vi "common_map_read.vi"(8 "error in":errorcluster, 11 "file path":path) -> (0 "error out":errorcluster, 3 "common map":map{string, T1}(c390))   [LabVIEW 2024, in "MemoryManager.lvclass"]
uses:
  MemoryManager.lvclass
  MemoryManager.lvclass/MemoryManager.ctl
  common_map_value--cluster.ctl
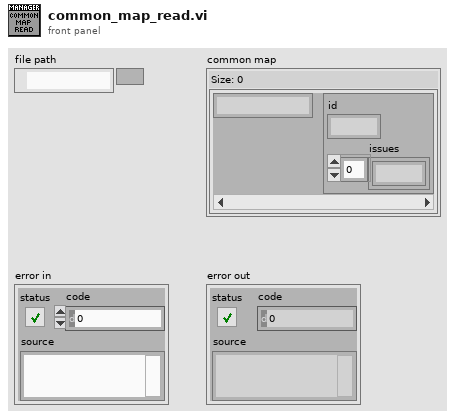
[diagram p1: front panel]
types:
  T1 = typedef "MemoryManager.lvclass/common_map_value--cluster.ctl" = cluster{"id":i32, "issues":i32[]}
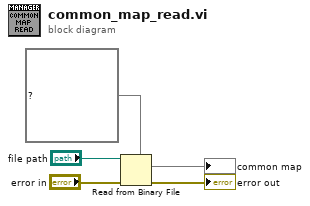
[diagram p0: block diagram]
diagram:
  n1 = Read from Binary File(5:map{string, T1} {} ("map"), 8:"error in", 11:"file path") -> (0:→"error out":errorcluster, 2:→"common map":map{string, T1})  [unwired: 3 in, 2 out]
